vi "WS1050 36 DUT CP CV Sweep F12_B1 SubVI.vi"(0 "TMN DC\\CAP Data Log File Path":path=path "C:/WS1050 36 DUT Data", 1 "Test Program":string="WS1050 36 DUT CP CV Sweep SubVI", 3 "Lot#":string="WS1050", 4 "Wafer#":string="T7-EB", 5 "Board#":string="BRD5", 6 "Temp":string, 7 "error in (no error)":errorcluster, 8 "File Name":string="CYC_WS1050_T7_EB_65C_40V_25DC_EMPTY_BRD5_141017_1", 9 "Comment":string="CYC65C40V", 10 "Ke2400":refnum<visa-resource-name>="GPIB0::3::INSTR", 11 "PS1 Source":refnum<visa-resource-name>="GPIB0::5::INSTR", 12 "Serial Number":string[][](table)=[["DUT", "SN"], ["DUT1", "1"], ["DUT2", "2"], ["DUT3", "3"], ["DUT4", "4"], ["DUT5", "5"], ["DUT6", "6"], ["DUT7", "7"], ["DUT8", "8"], ["DUT9", "9"], ["DUT10", "10"], ["DUT11", "11"], ["DUT12", "12"], ["DUT13", "13"], ["DUT14", "14"], ["DUT15", "15"], ["DUT16", "16"], ["DUT17", "17"], ["DUT18", "18"], ["DUT19", "19"], ["DUT20", "20"], ["DUT21", "21"], ["DUT22", "22"], ["DUT23", "23"], ["DUT24", "24"], ["DUT25", "25"], ["DUT26", "26"], ["DUT27", "27"], ["DUT28", "28"], ["DUT29", "29"], ["DUT30", "30"], ["DUT31", "31"], ["DUT32", "32"], ["DUT33", "33"], ["DUT34", "34"], ["DUT35", "35"], ["DUT36", "36"]], 14 "CP Set to Run":dbl[][](array[numeric]), 16 "HD/Cycles Completed":string="Test Data", 18 "Ke2000":refnum<visa-resource-name>="GPIB0::9::INSTR") -> (13 "40V_1":string[][](table), 15 "40V_2":string[][](table), 17 "40V_3":string[][](table), 20 "Plot_1":dbl[][](graph) caption="(Y) Multi Plot 2", 21 "Plot_2":dbl[][](graph) caption="(Y) Multi Plot 2", 22 "Ke2400 Out":refnum<visa-resource-name>="GPIB0::3::INSTR", 23 "Plot_3":dbl[][](graph) caption="(Y) Multi Plot 2", 24 "CP Voltage":string, 25 "PS1 Out":refnum<visa-resource-name>, 26 "Ke2000 Out":refnum<visa-resource-name>="GPIB0::9::INSTR", 27 "error out":errorcluster)   [LabVIEW 2012]
uses:
  WS_VCAP Driver 029/Source/WSVCAP Shell/Type Defs/WSVCAP SHL I2C DUT Mask Mode Enum.ctl
panel:
  in  "Reg1_Bit Cntrl":string[](array[string])=["01", "02", "04", "08", "10", "20", "40", "80", "03", "06", "0C", "D8", "33", "66", "CC", "07", "0E", "1C", "38", "70", "E0", "0F", "1E", "3C", "78", "F0", "1F", "3E", "7C", "F8", "3F", "7E", "FC", "7F", "FE", "FD", "FB", "F7", "EF", "DF", "BF", "7F", "FC", "F9", "F3", "E7", "CF", "9F", "3F", "F8", "F1", "E3", "C7", "8F", "1F", "F0", "E1", "C3", "87", "0F", "E0", "C1", "83", "07", "C0", "81", "03", "AA", "55", "00"]
  out "date string":string="5/19/2014"
  in  "VPI_Cmd":string[](array[string])=["00", "3B", "00"]
  in  "VPI Name":string[](array[string])=["All_Drivers OFF", "All Drivers ON", "All Drivers OFF2"]
  in  "Tab Control":T1(tab)
  in  "Set VDD":dbl=3.7 format="%.3g"
  in  "Clock Rate (Hz)":dbl=1000000.0 caption="Meas Speed" format="%.1p Hz"
  out "AR  Measurent(Hz)":dbl
  in  "RFFE Slave Address":u8=7 caption="Slave Address" format="0x%02x"
  in  "CP VPI":i32(ring) items=["CP HDC 35V", "CP HDC 40.25V", "CP HDC 27.5V", "CP HDC 30.5V", "CP HDC 44V"]
  in  "Control Panel":T2={"CP C-V \nSweep"=TRUE, "HD/CYC"=FALSE, "E-CAL"=FALSE, "DVA"=FALSE, "VPI"=FALSE, "VSA"=FALSE, "HS"=FALSE}
  out "CP C-V Sweep":bool
  out "HD/CYC":bool
  out "E-CAL":bool
  out "DVA":bool
  out "VPI":bool
  out "VSA":bool
  out "HS":bool
  in  "Freq(Hz)":string="12K"
  in  "Test Sequences":i32(ring) items=["C1_C2_C3", "C2_C1_C3", "C3_C2_C1"]
  in  "WS1050/51":bool=TRUE
  in  "CP with DVA ON":i32(ring) items=["CP HDC 35V", "CP HDC 40.25V", "CP HDC 27.5V", "CP HDC 30.5V", "CP HDC 44V"]
  in  "% Duty Cycle":string="NA"
  in  "Cmin/Act":bool=TRUE
  in  "Current Input":string="71.772763E+0"
  out "NOM IDD OFF(uA)":string
  out "No of HD/Cycle\nCompleted":i32
  out "Loop \ncompleted":i32=1
  out "Previous Time":string="12:20:26 PM"
  out "STATUS":string="Idle...."
  out "Total Delta C2(pF)":string[](array[string])
  out "Total Delta C1(pF)":string[](array[string])
  out "Total Delta C3(pF)":string[](array[string])
  out "RB Reg for HD/Cycle":string[](array[string])
  out "VPI C2":string[][](table)
  out "VPI C3":string[][](table)
  out "NOM IDD ON (uA)":string
  out "IDD_HD/CYC (uA)":string="164.601255E+0"
  out "IDD Stdby(uA)":string="2.606990E+0"
  out "VPI C1":string[][](table)
  out "Loops Run":i64
  out "VSA_V1":string[][](table)
  out "VSA_V2":string[][](table)
  out "VSA_V3":string[][](table)
  in  "VSA Voltage(V)":dbl[](array[numeric])=[-10.0, 0.0, 10.0]
  in  "X Repeat":i32=100
  out "% Delta C_T0":string[][](array[string])
  out "% Delta C":string[][](array[string])
  out "EFuse RB T0":string[](array[string])
  out "Current EFuse Read back":string[](array[string])
  out "EFuse Readback Status":bool[](array[boolean])
  in  "DeltaC Target Setting(pF)":dbl=7.375
  in  "Debug":bool
  in  "No of Rows\nFrom Spread Sheet":i32
  in  "Plot Delta Cmin":bool=TRUE
  in  "Plot":T3(ring)
  in  "Bank1":i32(ring)=6 items=["C1", "C2", "C3", "D_C1", "D_C2", "D_C3", "D_B1_C1", "D_B1_C2", "D_B1_C3"]
  in  "Bank2":i32(ring)=7 items=["C1", "C2", "C3", "D_C1", "D_C2", "D_C3", "D_B1_C1", "D_B1_C2", "D_B1_C3"]
  in  "Bank3":i32(ring)=8 items=["C1", "C2", "C3", "D_C1", "D_C2", "D_C3", "D_B1_C1", "D_B1_C2", "D_B1_C3"]
  # "Company:  WiSpry Inc\n20 Fairbanks Ste 198 Irvine CA 92618\n\nAuthor:  Andy V Tran\nCreated:  08/21/2015\nLabVIEW 2012 Pro\nTest Program:  WS1050 36 DUT CP CV Sweep SubVI\nFPGA: WS_VCAP Driver 029"
  # "Note for HD Duty Cycle:\n1.  Set time to start HD_DC (Min), default is 259200 (6 months) \n2.  Set Time for Duty Cycle ON/OFF, default setting is 2 minutes\n3.  No of Loops to RP = 3600s/(Time ALL ON(s) + Time ALL + OFF(s))\n4.  Set X Repeat = no of runs, default is 100 runs\n5.  Set TTF Completed to stop the test.\n\nVer 1.1 updated based on Ver1.0:\n1.  Updated the control panel ( CP C-V Sweep was set \"Yes\" by default)\n2.  CP Voltage sweep should be set up from look up table."
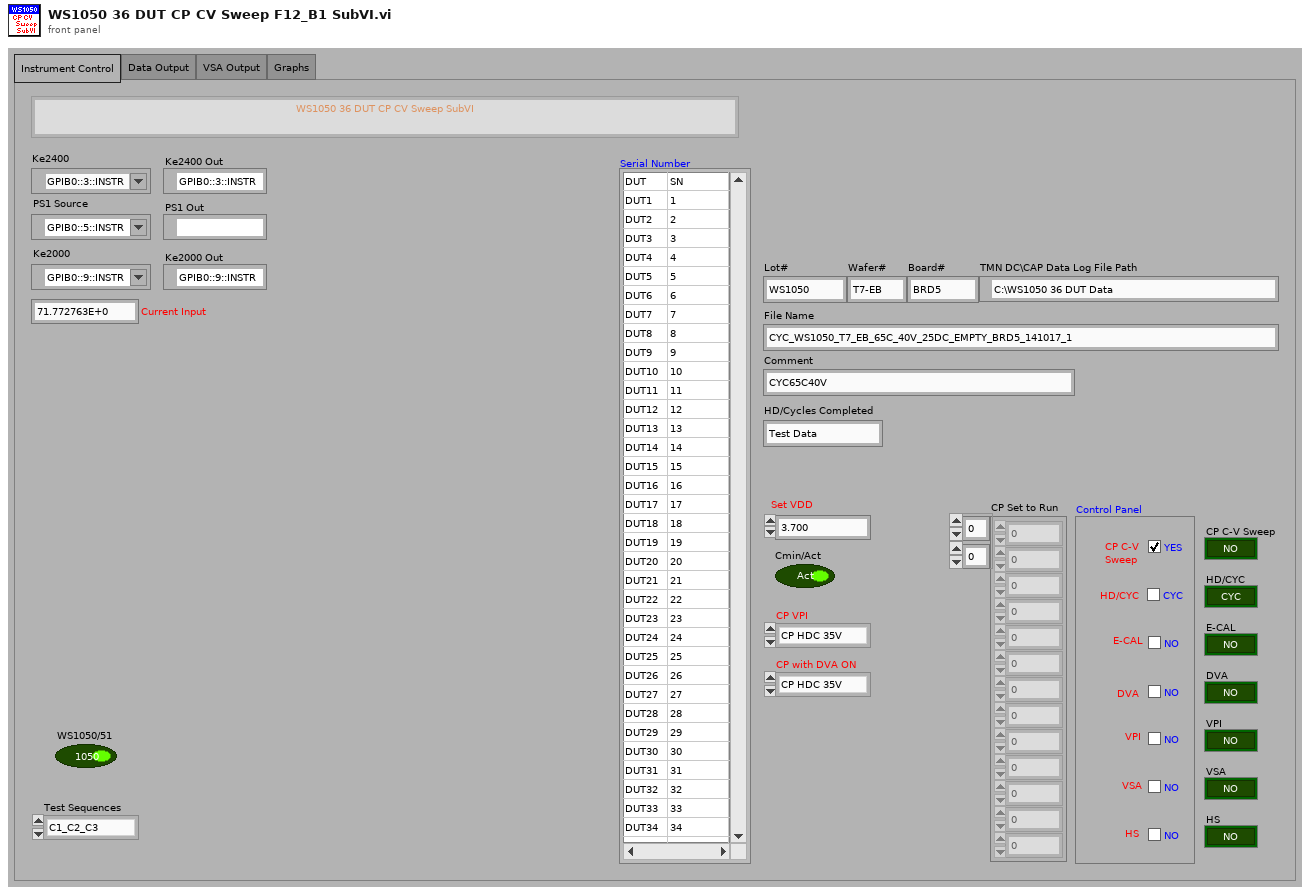
[diagram p1: front panel]
types:
  T1 = enum32{"Instrument Control", "Data Output", "VSA Output", "Graphs"}
  T2 = cluster{"CP C-V \nSweep":bool, "HD/CYC":bool, "E-CAL":bool, "DVA":bool, "VPI":bool, "VSA":bool, "HS":bool}
  T3 = enum16{"ALL DUTs", "DUT 01", "DUT 02", "DUT 03", "DUT 04", "DUT 05", "DUT 06", "DUT 07", "DUT 08", "DUT 09", "DUT 10", "DUT 11", "DUT 12", "DUT 13", "DUT 14", "DUT 15", "DUT 16", "DUT 17", "DUT 18", "DUT 19", "DUT 20", "DUT 21", "DUT 22", "DUT 23", "DUT 24", "DUT 25", "DUT 26", "DUT 27", "DUT 28", "DUT 29", "DUT 30", "DUT 31", "DUT 32", "DUT 33", "DUT 34", "DUT 35", "DUT 36"}
  T4 = typedef "WSVCAP SHL I2C DUT Mask Mode Enum.ctl" = enum16{"Custom", "C1", "C2", "C3", "All"}
  T5 = cluster{"Test Program ":string, "Comment":string, "Data Out":string, "Data Out":string, "CP Voltage":string, string, "% Duty Cycle":string, "CP Voltage":string, "string":string, "Freq(Hz)":string, "Board#":string}
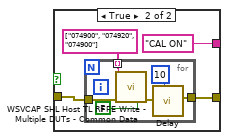
[diagram p3: hidden frame]
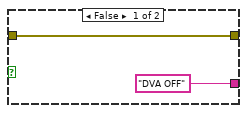
[diagram p4: hidden frame]
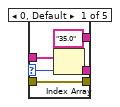
[diagram p5: hidden frame]
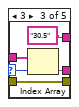
[diagram p6: hidden frame]
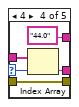
[diagram p7: hidden frame]
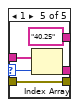
[diagram p8: hidden frame]
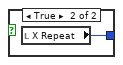
[diagram p9: hidden frame]
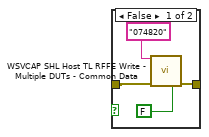
[diagram p10: hidden frame]
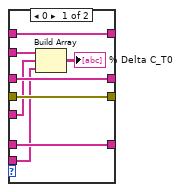
[diagram p11: hidden frame]
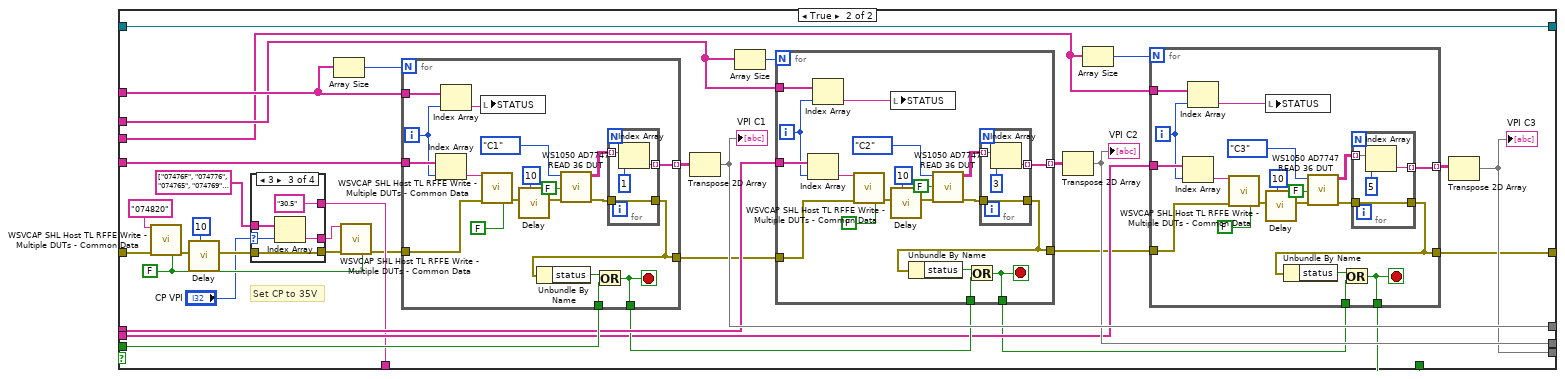
[diagram p12: hidden frame]
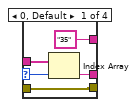
[diagram p13: hidden frame]
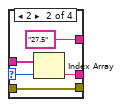
[diagram p14: hidden frame]
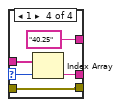
[diagram p15: hidden frame]
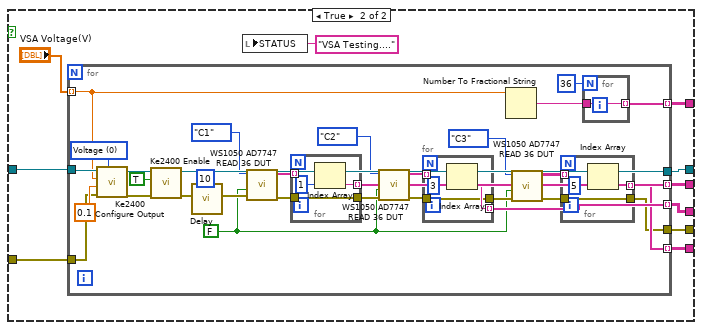
[diagram p17: hidden frame]
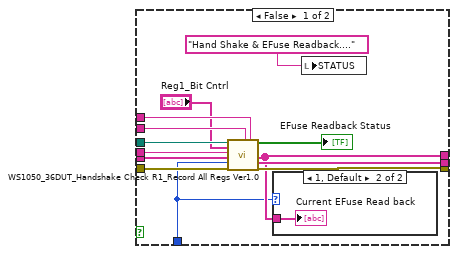
[diagram p18: hidden frame]
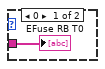
[diagram p19: hidden frame]
diagram:
  n1 = call "WSVCAP SHL Host TL RFFE Configure.vi"("RFFE Slave Address"="RFFE Slave Address", "Clock Rate (Hz)"="Clock Rate (Hz)", "error in"="error in (no error)") -> ("error out"=w4:errorcluster)  [unwired: 11 in, 1 out]
  n2 = call "Control Panel.vi"("error in (no error)"=w4, "Control Panel"="Control Panel") -> ("error out"=w12:errorcluster, "VPI"=w8:bool, "DVA"=w9:bool, "E-CAL"=w10:bool, "VSA"=w7:bool, "HD/CYC"=w11:bool, "HS"=w6:bool, "Verify Socket"=w1:bool)  [unwired: 2 in]
  "CP C-V Sweep" <- w1
  "E-CAL" <- w10
  "VPI" <- w8
  "VSA" <- w7
  "HS" <- w6
  "HD/CYC" <- w11
  "DVA" <- w9
  n3 = case shown="True" w1 {
    tunnel: w12 -> [w26 w28]
    tunnel: [w26 w32] -> w15
    tunnel: "CP Set to Run" -> [_ w76]
    tunnel: "PS1 Source" -> [w24 w29]
    tunnel: "Ke2000" -> [w25 w72]
    tunnel: [w25 w75] -> w22
    tunnel: [w24 w33] -> w21
    tunnel: "Ke2400" -> [w23 w69]
    tunnel: [w23 w66] -> w16
    tunnel: "RFFE Slave Address" -> [_ w64]
    tunnel: w11 -> [_ w43]
    tunnel: w10 -> [_ w42]
    tunnel: w9 -> [_ w27]
    tunnel: w8 -> [_ w41]
    tunnel: w7 -> [_ w40]
    tunnel: w6 -> [_ w39]
    tunnel: "Clock Rate (Hz)" -> [_ w31]
    frame False {
    }
    frame True {
      w30 = u32 1 ("milliseconds to wait")
      # "VSA"
      # "HS"
      # "HD/CYC"
      # "DVA"
      # "E-CAL"
      # "VPI"
      n4 = call "WSVCAP SHL Host TL RFFE Write - Multiple DUTs - Common Data.vi"("Data Out"="074000", "error in"=w28, "Log (T)"=FALSE) -> ("error out"=w74:errorcluster)  [unwired: 12 in]
      n5 = call "Delay.vi"("milliseconds to wait"=u32 100, "error in (no error)"=w74) -> ("error out"=w73:errorcluster)  [unwired: 9 in]
      n6 = call "Ke2000 Single Reading.vi"("error in (no error)"=w73, "VISA resource name"=w72) -> ("error out"=w54:errorcluster, "VISA resource name out"=w71:refnum<visa-resource-name>, "uA"=w56:string)  [unwired: 5 in, 2 out]
      n7 = call "Substration.vi"("error in (no error)"=w54, "Input2"="Current Input", "Input1"=w56) -> ("error out"=w36:errorcluster, "In1 - In2"=w55:string)  [unwired: 7 in]
      "IDD Stdby(uA)" <- w55
      n8 = case shown="False" w43 {
        tunnel: [1 ("X Repeat") w133] -> w65
        frame False {
        }
        frame True {
          n9 = local read "X Repeat"() -> (w133:i32)
        }
      }
      n10 = call "WSVCAP SHL Host TL RFFE Write - Multiple DUTs - Common Data.vi"("Data Out"="074040", "error in"=w36, "Log (T)"=FALSE) -> ("error out"=w35:errorcluster)  [unwired: 12 in]
      n11 = call "Delay.vi"("milliseconds to wait"=w30, "error in (no error)"=w35) -> ("error out"=w62:errorcluster)  [unwired: 9 in]
      n12 = case shown="True" w27 {
        tunnel: w62 -> [w94 w104]
        tunnel: [w94 w102] -> w60
        tunnel: ["DVA OFF" ("Data Out") "DVA ON" ("Data Out")] -> w61
        frame False {
        }
        frame True {
          n13 = call "WSVCAP SHL Host TL RFFE Write - Multiple DUTs - Common Data.vi"("Data Out"="074800", "error in"=w104, "Log (T)"=FALSE) -> ("error out"=w100:errorcluster)  [unwired: 12 in]
          n14 = case shown="2" "CP with DVA ON" {
            selector: "CP with DVA ON" -> [w110 w115 w120 w125 w129]
            tunnel: string[] ["07442F", "074436", "074428", "074429", "07443B"] -> [w111 w116 w121 w126 w131]
            tunnel: [w109 w114 w119 w124 w130] -> w96
            tunnel: ["35.0" ("Data Out") "29.75" ("Data Out") "30.5" ("Data Out") "44.0" ("Data Out") "40.25" ("Data Out")] -> _
            tunnel: w100 -> [w107 w112 w117 w122 w127]
            tunnel: [w107 w112 w117 w122 w127] -> w99
            frame 0, Default {
              n15 = Index Array(array=w111, index=w110) -> (element=w109:string)
            }
            frame 2 {
              n16 = Index Array(array=w116, index=w115) -> (element=w114:string)
            }
            frame 3 {
              n17 = Index Array(array=w121, index=w120) -> (element=w119:string)
            }
            frame 4 {
              n18 = Index Array(array=w126, index=w125) -> (element=w124:string)
            }
            frame 1 {
              n19 = Index Array(array=w131, index=w129) -> (element=w130:string)
            }
          }
          n20 = call "WSVCAP SHL Host TL RFFE Write - Multiple DUTs - Common Data.vi"("Data Out"=w96, "error in"=w99, "Log (T)"=FALSE) -> ("error out"=w102:errorcluster)  [unwired: 12 in]
        }
      }
      n21 = for {
        N: 36 -> [_]
        tunnel: "Serial Number" -> [w81]
        tunnel: [w79] -> w45 mode=indexing
        i -> [w78]
        n22 = Increment(x=w78) -> (x+1=w77:i32)
        n23 = Index Array(array=w81, index (row)=w77, index (col)=1 ("disabled index (col)")) -> (element=w79:string)
      }
      n24 = Not(x=w39) -> (.not. x?=w44:bool)
      n25 = Number To Fractional String(number="Set VDD", precision (6)=i16 2) -> (F-format string=w58:string)  [unwired: 2 in]
      n26 = call "Delay.vi"("milliseconds to wait"=w30, "error in (no error)"=w60) -> ("error out"=w51:errorcluster)  [unwired: 9 in]
      n27 = case shown="False" w42 {
        tunnel: w51 -> [w82 w85]
        tunnel: [w82 w84] -> w50
        tunnel: ["CAL OFF" ("Data Out") "CAL ON" ("Data Out")] -> w52
        frame False {
        }
        frame True {
          n28 = for {
            tunnel: string[] ["074900", "074920", "074900"] -> [w93] mode=indexing
            tunnel: w85 -> [w90]
            tunnel: [w89] -> w84
            n29 = call "WSVCAP SHL Host TL RFFE Write - Multiple DUTs - Common Data.vi"("Data Out"=w93, "error in"=w90, "Log (T)"=FALSE) -> ("error out"=w92:errorcluster)  [unwired: 12 in]
            n30 = call "Delay.vi"("milliseconds to wait"=u32 10, "error in (no error)"=w92) -> ("error out"=w89:errorcluster)  [unwired: 9 in]
          }
        }
      }
      n31 = for {
        N: w65 -> [_]
        tunnel: w76 -> [w162]
        tunnel: [w158] -> w75
        tunnel: w55 -> [w157]
        tunnel: w71 -> [w156]
        tunnel: "TMN DC\\CAP Data Log File Path" -> [w155]
        tunnel: w69 -> [w153]
        tunnel: [w152] -> w67
        tunnel: w29 -> [w137]
        tunnel: w64 -> [w148]
        tunnel: w61 -> [w147]
        tunnel: w58 -> [w146]
        tunnel: [w145] -> w53
        tunnel: w52 -> [w144]
        tunnel: w50 -> [w143]
        tunnel: w27 -> [w142]
        tunnel: w41 -> [w141]
        tunnel: w44 -> [w140]
        tunnel: w40 -> [w139]
        tunnel: w45 -> [w138]
        tunnel: [w137] -> w33
        tunnel: "Current Input" -> [w136]
        tunnel: w31 -> [w134]
        stop <- w135 stop-if-true
        (unwired) u64 0
        n32 = while {
          tunnel: w162 -> [w180]
          tunnel: w155 -> [w381]
          tunnel: "Lot#" -> [w380]
          tunnel: "Wafer#" -> [w379]
          tunnel: w138 -> [w378]
          tunnel: "Test Program" -> [w377]
          tunnel: w138 -> [w376]
          tunnel: "Comment" -> [w375]
          tunnel: "Lot#" -> [w374]
          tunnel: "Wafer#" -> [w373]
          tunnel: w156 -> [w370]
          tunnel: [w372] -> w158
          tunnel: w157 -> [w369]
          tunnel: w153 -> [w367]
          tunnel: [w366] -> w152
          tunnel: [w291] -> w149
          tunnel: w148 -> [w290]
          tunnel: w147 -> [w240]
          tunnel: w146 -> [w238]
          tunnel: [w220] -> w145
          tunnel: w144 -> [w225]
          tunnel: w143 -> [w181]
          tunnel: w142 -> [w224]
          tunnel: w141 -> [w217]
          tunnel: w140 -> [w212]
          tunnel: w139 -> [w206]
          tunnel: w136 -> [w166]
          tunnel: w134 -> [w165]
          i -> [w185]
          stop <- w320 stop-if-true
          n33 = Array Size(array=w180) -> (size(s)=w179:i32[])
          n34 = Index Array(array=w180, index (row)=w185, index (col)=0 ("disabled index (col)")) -> (element=w177:dbl)
          n35 = Index Array(array=w179, index=0) -> (element=w168:i32)
          n36 = call "CP_Cmd_Setting.vi"("error in (no error)"=w181, "Input"=w177) -> ("error out"=w184:errorcluster, "CP Voltage"=w182:string, "Send Cmd"=w183:string)  [unwired: 6 in, 1 out]
          "CP Voltage" <- w182
          n37 = To Quad Integer(1:w168) -> (0:w167:i64)
          n38 = flat-sequence {
            tunnel: [w434] -> w365
            tunnel: w370 -> [w423]
            tunnel: w369 -> [w435]
            tunnel: [w435] -> w364
            tunnel: [w400] -> w363
            tunnel: [w397] -> w362
            tunnel: w184 -> [w432]
            tunnel: w185 -> [w382]
            tunnel: [w382] -> w319
            tunnel: ["Temp"] -> w314
            tunnel: [w405] -> w309
            tunnel: [w404] -> w308
            tunnel: [w403] -> w307
            tunnel: [w409] -> w297
            tunnel: [w406] -> w296
            tunnel: w290 -> [w431]
            tunnel: [w431] -> w289
            tunnel: [w408] -> w277
            tunnel: [w407] -> w253
            tunnel: [w383] -> w241
            tunnel: w183 -> [w429]
            tunnel: ["% Duty Cycle"] -> w237
            tunnel: [w390] -> w229
            tunnel: w217 -> [w418]
            tunnel: [w418] -> w216
            tunnel: w212 -> [w417]
            tunnel: [w417] -> w211
            tunnel: w206 -> [w416]
            tunnel: [w416] -> w205
            tunnel: [w412] -> w200
            tunnel: ["WS1050/51"] -> w194
            tunnel: ["Cmin/Act"] -> w190
            tunnel: w167 -> [w388]
            tunnel: w177 -> [w389]
            tunnel: [w388] -> w176
            tunnel: w166 -> [w387]
            tunnel: w165 -> [w383]
            tunnel: [w487] -> w288
            tunnel: w365 -> [w490]
            tunnel: w364 -> [w493]
            tunnel: w363 -> [w489]
            tunnel: w362 -> [w488]
            tunnel: [w478] -> w287
            tunnel: [w493] -> w286
            tunnel: [w489] -> w285
            tunnel: [w488] -> w284
            tunnel: w319 -> [w492]
            tunnel: [w492] -> w283
            tunnel: w314 -> [w491]
            tunnel: [w491] -> w282
            tunnel: [w490] -> w281
            tunnel: w309 -> [w486]
            tunnel: w308 -> [w471]
            tunnel: w307 -> [w472]
            tunnel: [w483] -> w280
            tunnel: w297 -> [w485]
            tunnel: w296 -> [w483]
            tunnel: [w479] -> w279
            tunnel: w289 -> [w484]
            tunnel: [w469] -> w278
            tunnel: w277 -> [w469]
            tunnel: [w471] -> w276
            tunnel: w253 -> [w470]
            tunnel: [w470] -> w252
            tunnel: [w472] -> w250
            tunnel: w241 -> [w482]
            tunnel: [w481] -> w230
            tunnel: w229 -> [w481]
            tunnel: w216 -> [w477]
            tunnel: [w477] -> w215
            tunnel: w211 -> [w476]
            tunnel: [w476] -> w210
            tunnel: w205 -> [w475]
            tunnel: [w475] -> w204
            tunnel: w200 -> [w474]
            tunnel: [w473] -> w199
            tunnel: w194 -> [w467]
            tunnel: [w467] -> w193
            tunnel: w190 -> [w466]
            tunnel: [w466] -> w189
            tunnel: w176 -> [w465]
            tunnel: [w465] -> w175
            tunnel: w288 -> [w532]
            tunnel: [w531] -> w275
            tunnel: w287 -> [w523]
            tunnel: [w523] -> w272
            tunnel: w286 -> [w542]
            tunnel: [w542] -> w270
            tunnel: w285 -> [w541]
            tunnel: [w541] -> w268
            tunnel: w284 -> [w540]
            tunnel: [w540] -> w266
            tunnel: w283 -> [w539]
            tunnel: [w539] -> w264
            tunnel: w282 -> [w538]
            tunnel: [w538] -> w262
            tunnel: w281 -> [w537]
            tunnel: [w537] -> w260
            tunnel: w280 -> [w536]
            tunnel: [w536] -> w258
            tunnel: [w528] -> w256
            tunnel: w279 -> [w527]
            tunnel: w278 -> [w534]
            tunnel: w276 -> [w533]
            tunnel: w252 -> [w520]
            tunnel: [w520] -> w251
            tunnel: w250 -> [w522]
            tunnel: [w522] -> w249
            tunnel: [w529] -> w248
            tunnel: [w530] -> w231
            tunnel: w230 -> [w530]
            tunnel: w215 -> [w526]
            tunnel: [w526] -> w214
            tunnel: w210 -> [w525]
            tunnel: [w525] -> w209
            tunnel: w204 -> [w524]
            tunnel: [w524] -> w203
            tunnel: w199 -> [w521]
            tunnel: [w521] -> w196
            tunnel: w193 -> [w518]
            tunnel: [w518] -> w192
            tunnel: w189 -> [w517]
            tunnel: [w517] -> w188
            tunnel: w175 -> [w516]
            tunnel: [w516] -> w174
            tunnel: w275 -> [w582]
            tunnel: [w581] -> w274
            tunnel: [w577] -> w273
            tunnel: w272 -> [w571]
            tunnel: [w571] -> w271
            tunnel: w270 -> [w593]
            tunnel: [w593] -> w269
            tunnel: w268 -> [w592]
            tunnel: [w592] -> w267
            tunnel: w266 -> [w591]
            tunnel: [w591] -> w265
            tunnel: w264 -> [w590]
            tunnel: [w590] -> w263
            tunnel: w262 -> [w589]
            tunnel: [w589] -> w261
            tunnel: w260 -> [w588]
            tunnel: [w588] -> w259
            tunnel: w258 -> [w587]
            tunnel: [w587] -> w257
            tunnel: w256 -> [w586]
            tunnel: [w586] -> w255
            tunnel: [w569] -> w254
            tunnel: w251 -> [w584]
            tunnel: w249 -> [w583]
            tunnel: w248 -> [w576]
            tunnel: ["DeltaC Target Setting(pF)"] -> w239
            tunnel: [w579] -> w232
            tunnel: w231 -> [w579]
            tunnel: w224 -> [w578]
            tunnel: [w578] -> w223
            tunnel: w214 -> [w575]
            tunnel: [w575] -> w213
            tunnel: w209 -> [w574]
            tunnel: [w574] -> w208
            tunnel: w203 -> [w573]
            tunnel: [w573] -> w202
            tunnel: w196 -> [w572]
            tunnel: [w569] -> w195
            tunnel: w192 -> [w568]
            tunnel: [w568] -> w191
            tunnel: w188 -> [w567]
            tunnel: [w567] -> w187
            tunnel: w174 -> [w566]
            tunnel: [w566] -> w173
            tunnel: [w671] -> w361
            tunnel: [w640] -> w360
            tunnel: w274 -> [w674]
            tunnel: w273 -> [w651]
            tunnel: [w660] -> w359
            tunnel: [w651] -> w358
            tunnel: [w673] -> w357
            tunnel: [w672] -> w356
            tunnel: w271 -> [w660]
            tunnel: w269 -> [w670]
            tunnel: [w670] -> w355
            tunnel: w267 -> [w666]
            tunnel: [w666] -> w354
            tunnel: w265 -> [w665]
            tunnel: [w665] -> w353
            tunnel: w263 -> [w661]
            tunnel: [w661] -> w318
            tunnel: w261 -> [w669]
            tunnel: [w669] -> w313
            tunnel: w259 -> [w668]
            tunnel: [w667] -> w310
            tunnel: w257 -> [w663]
            tunnel: w255 -> [w659]
            tunnel: [w664] -> w306
            tunnel: [w662] -> w305
            tunnel: [w659] -> w300
            tunnel: w254 -> [w658]
            tunnel: [w648] -> w295
            tunnel: [w647] -> w294
            tunnel: [w646] -> w293
            tunnel: w239 -> [w657]
            tunnel: [w645] -> w233
            tunnel: w232 -> [w645]
            tunnel: [w644] -> w228
            tunnel: w223 -> [w643]
            tunnel: w213 -> [w638]
            tunnel: w208 -> [w637]
            tunnel: [w637] -> w207
            tunnel: w202 -> [w636]
            tunnel: [w636] -> w201
            tunnel: w195 -> [w633]
            tunnel: w191 -> [w632]
            tunnel: w187 -> [w621]
            tunnel: w173 -> [w620]
            tunnel: [w620] -> w172
            tunnel: w361 -> [w877]
            tunnel: [w877] -> w352
            tunnel: [w863] -> w351
            tunnel: [w876] -> w350
            tunnel: w360 -> [w875]
            tunnel: w359 -> [w874]
            tunnel: w358 -> [w873]
            tunnel: [w874] -> w349
            tunnel: [w873] -> w348
            tunnel: w357 -> [w872]
            tunnel: [w872] -> w347
            tunnel: w356 -> [w871]
            tunnel: [w871] -> w346
            tunnel: w355 -> [w870]
            tunnel: [w870] -> w345
            tunnel: w354 -> [w869]
            tunnel: [w869] -> w344
            tunnel: w353 -> [w868]
            tunnel: [w868] -> w343
            tunnel: w367 -> [w867]
            tunnel: [w865] -> w342
            tunnel: [w845] -> w341
            tunnel: [w846] -> w340
            tunnel: [w844] -> w339
            tunnel: w318 -> [w861]
            tunnel: [w861] -> w317
            tunnel: w313 -> [w860]
            tunnel: [w860] -> w312
            tunnel: w310 -> [w876]
            tunnel: w306 -> [w858]
            tunnel: w305 -> [w859]
            tunnel: [w859] -> w304
            tunnel: [w858] -> w302
            tunnel: w300 -> [w857]
            tunnel: [w857] -> w299
            tunnel: w295 -> [w843]
            tunnel: w294 -> [w842]
            tunnel: w293 -> [w841]
            tunnel: [w838] -> w292
            tunnel: [w843] -> w247
            tunnel: [w842] -> w245
            tunnel: [w841] -> w243
            tunnel: [w840] -> w234
            tunnel: w233 -> [w840]
            tunnel: w228 -> [w839]
            tunnel: [w839] -> w227
            tunnel: w207 -> [w838]
            tunnel: w201 -> [w837]
            tunnel: w172 -> [w836]
            tunnel: [w836] -> w171
            tunnel: w352 -> [w971]
            tunnel: [w971] -> w338
            tunnel: w351 -> [w992]
            tunnel: [w991] -> w337
            tunnel: w381 -> [w993]
            tunnel: w380 -> [w990]
            tunnel: w379 -> [w989]
            tunnel: w378 -> [w988]
            tunnel: [w987] -> w336
            tunnel: w350 -> [w981]
            tunnel: [w981] -> w335
            tunnel: w349 -> [w986]
            tunnel: w348 -> [w985]
            tunnel: [w986] -> w334
            tunnel: [w985] -> w333
            tunnel: [w979] -> w332
            tunnel: w347 -> [w984]
            tunnel: [w984] -> w331
            tunnel: w346 -> [w983]
            tunnel: [w983] -> w330
            tunnel: [w982] -> w329
            tunnel: w345 -> [w980]
            tunnel: w344 -> [w978]
            tunnel: w343 -> [w977]
            tunnel: "File Name" -> [w976]
            tunnel: w342 -> [w975]
            tunnel: [w975] -> w328
            tunnel: w341 -> [w974]
            tunnel: [w974] -> w327
            tunnel: [w973] -> w326
            tunnel: w340 -> [w973]
            tunnel: w339 -> [w972]
            tunnel: [w972] -> w325
            tunnel: w317 -> [w955]
            tunnel: [w955] -> w315
            tunnel: w312 -> [w969]
            tunnel: [w969] -> w311
            tunnel: w304 -> [w968]
            tunnel: [w968] -> w303
            tunnel: w302 -> [w967]
            tunnel: [w967] -> w301
            tunnel: w299 -> [w966]
            tunnel: [w966] -> w298
            tunnel: w292 -> [w965]
            tunnel: w247 -> [w964]
            tunnel: [w964] -> w246
            tunnel: w245 -> [w963]
            tunnel: [w963] -> w244
            tunnel: w243 -> [w962]
            tunnel: [w962] -> w242
            tunnel: w237 -> [w961]
            tunnel: [w961] -> w236
            tunnel: [w960] -> w235
            tunnel: w234 -> [w960]
            tunnel: w227 -> [w959]
            tunnel: [w959] -> w226
            tunnel: ["Freq(Hz)"] -> w198
            tunnel: ["Board#"] -> w197
            tunnel: w171 -> [w956]
            tunnel: [w956] -> w170
            tunnel: ["Debug"] -> w164
            tunnel: w338 -> [w1066]
            tunnel: w337 -> [w1065]
            tunnel: w381 -> [w1032]
            tunnel: w377 -> [w1060]
            tunnel: w376 -> [w1063]
            tunnel: w375 -> [w1059]
            tunnel: w374 -> [w1062]
            tunnel: w373 -> [w1058]
            tunnel: w336 -> [w1061]
            tunnel: [w1066] -> w322
            tunnel: [w1064] -> w323
            tunnel: w335 -> [w1056]
            tunnel: [w1056] -> w324
            tunnel: w334 -> [w1055]
            tunnel: w333 -> [w1043]
            tunnel: w332 -> [w1054]
            tunnel: w331 -> [w1053]
            tunnel: w330 -> [w1045]
            tunnel: w329 -> [w1052]
            tunnel: "File Name" -> [w1026]
            tunnel: w328 -> [w1051]
            tunnel: [w1051] -> w321
            tunnel: w327 -> [w1050]
            tunnel: w326 -> [w1049]
            tunnel: w325 -> [w1048]
            tunnel: [w1028] -> w316
            tunnel: w315 -> [w1028]
            tunnel: w311 -> [w1047]
            tunnel: w303 -> [w1046]
            tunnel: w301 -> [w1044]
            tunnel: w298 -> [w1015]
            tunnel: w246 -> [w1042]
            tunnel: w244 -> [w1041]
            tunnel: w242 -> [w1040]
            tunnel: w240 -> [w1039]
            tunnel: w225 -> [w1038]
            tunnel: w182 -> [w1037]
            tunnel: w238 -> [w1036]
            tunnel: w236 -> [w1035]
            tunnel: w235 -> [w1034]
            tunnel: w226 -> [w1033]
            tunnel: [w1030] -> w222
            tunnel: [w1023] -> w218
            tunnel: w198 -> [w1022]
            tunnel: w197 -> [w1020]
            tunnel: w170 -> [w1019]
            tunnel: [w1019] -> w169
            tunnel: w164 -> [w1017]
            tunnel: [w1085] -> w371
            tunnel: [w1086] -> w372
            tunnel: [w1087] -> w291
            tunnel: w324 -> [w1086]
            tunnel: w323 -> [w1079]
            tunnel: w322 -> [w1087]
            tunnel: w321 -> [w1080]
            tunnel: [w1080] -> w366
            tunnel: w316 -> [w1072]
            tunnel: [w1078] -> w219
            tunnel: w222 -> [w1077]
            tunnel: w218 -> [w1075]
            tunnel: w169 -> [w1074]
            tunnel: [w1071] -> w163
            frame #0 {
              w413 = FALSE ("Log (T)")
              n39 = call "WSVCAP SHL Host TL RFFE Write - Multiple DUTs - Common Data.vi"("Data Out"=w429, "error in"=w432, "Log (T)"=FALSE) -> ("error out"=w419:errorcluster)  [unwired: 12 in]
              n40 = for {
                tunnel: string[] ["0760", "0767", "0768"] -> [w457] mode=indexing
                tunnel: [w453] -> w421 mode=indexing
                tunnel: w419 -> [w451]
                tunnel: [w450] -> w420
                i -> [w456]
                n41 = call "Delay.vi"("milliseconds to wait"=u32 10, "error in (no error)"=w451) -> ("error out"=w458:errorcluster)  [unwired: 9 in]
                n42 = call "WSVCAP SHL Host TL RFFE Read - Multiple DUTs - Common Data.vi"("Data Out"=w457, "error in"=w458, "Log (T)"=FALSE) -> ("RFFE Data In"=w455:string[], "error out"=w450:errorcluster)  [unwired: 11 in]
                n43 = Index Array(array=w455, index=w456) -> (element=w452:string)
                n44 = String Subset(string=w452, offset (0)=0) -> (substring=w453:string)  [unwired: 1 in]
              }
              "RB Reg for HD/Cycle" <- w421
              n45 = call "Delay.vi"("milliseconds to wait"=u32 100, "error in (no error)"=w420) -> ("error out"=w425:errorcluster)  [unwired: 9 in]
              n46 = call "Ke2000 Single Reading.vi"("error in (no error)"=w425, "VISA resource name"=w423) -> ("error out"=w427:errorcluster, "VISA resource name out"=w402:refnum<visa-resource-name>, "uA"=w428:string)  [unwired: 5 in, 2 out]
              n47 = call "Substration.vi"("error in (no error)"=w427, "Input2"=w387, "Input1"=w428) -> ("error out"=w384:errorcluster, "In1 - In2"=→"IDD_HD/CYC (uA)":string)  [unwired: 7 in]
              n48 = call "CP_Cmd_Setting.vi"("error in (no error)"=w384, "Input"=w389) -> ("error out"=w392:errorcluster, "CP Voltage"=w390:string, "Send Cmd"=w391:string)  [unwired: 6 in, 1 out]
              n49 = call "WSVCAP SHL Host TL RFFE Write - Multiple DUTs - Common Data.vi"("Data Out"=w391, "error in"=w392, "Log (T)"=w413) -> ("error out"=w430:errorcluster)  [unwired: 12 in]
              n50 = flat-sequence {
                tunnel: w415 -> [w460]
                tunnel: [w460] -> w411
                frame #0 {
                  w461 = "0" ("NOM IDD OFF(uA)")
                  w462 = string[] []
                  w463 = string[][] []
                  n51 = local write "Total Delta C1(pF)"(w462) -> ()
                  n52 = local write "Total Delta C2(pF)"(w462) -> ()
                  n53 = local write "Total Delta C3(pF)"(w462) -> ()
                  n54 = local write "Current EFuse Read back"(w462) -> ()
                  n55 = local write "NOM IDD ON (uA)"(w461) -> ()
                  n56 = local write "NOM IDD OFF(uA)"(w461) -> ()
                  n57 = local write "VSA_V3"(w463) -> ()
                  n58 = local write "VSA_V1"(w463) -> ()
                  n59 = local write "VSA_V2"(w463) -> ()
                  n60 = local write "VPI C1"(w463) -> ()
                  n61 = local write "VPI C2"(w463) -> ()
                  n62 = local write "VPI C3"(w463) -> ()
                  n63 = local write "% Delta C"(w463) -> ()
                  n64 = local write "40V_3"(w463) -> ()
                  n65 = local write "40V_2"(w463) -> ()
                  n66 = local write "40V_1"(w463) -> ()
                }
              }
              n67 = call "Delay.vi"("milliseconds to wait"=u32 10, "error in (no error)"=w430) -> ("error out"=w395:errorcluster)  [unwired: 9 in]
              n68 = for {
                tunnel: [w448] -> w434
                tunnel: [w447] -> w415
                tunnel: w413 -> [w446]
                tunnel: w402 -> [w445]
                tunnel: w395 -> [w441]
                tunnel: string[] ["0702013B3B3B", "070201000000"] -> [w438] mode=indexing
                tunnel: [w437] -> w398 mode=indexing
                tunnel: w387 -> [w436]
                n69 = call "WSVCAP SHL Host TL RFFE Write - Multiple DUTs - Common Data.vi"("Data Out"=w438, "error in"=w441, "Log (T)"=w446) -> ("error out"=w442:errorcluster)  [unwired: 12 in]
                n70 = call "Delay.vi"("milliseconds to wait"=u32 100, "error in (no error)"=w442) -> ("error out"=w443:errorcluster)  [unwired: 9 in]
                n71 = call "Ke2000 Single Reading.vi"("error in (no error)"=w443, "VISA resource name"=w445) -> ("error out"=w440:errorcluster, "VISA resource name out"=w448:refnum<visa-resource-name>, "uA"=w439:string)  [unwired: 5 in, 2 out]
                n72 = call "Substration.vi"("error in (no error)"=w440, "Input2"=w436, "Input1"=w439) -> ("error out"=w447:errorcluster, "In1 - In2"=w437:string)  [unwired: 7 in]
              }
              n73 = Index Array(array=w398, index=0) -> (element=w400:string)
              n74 = Index Array(array=w398, index=1) -> (element=w397:string)
              n75 = call "Multi Dut Cmd_Header Setting F12_B1.vi"("WS1050/51"="WS1050/51", "Cmin/Act"="Cmin/Act", "Test Seq"="Test Sequences", "error in (no error)"=w411) -> ("Name 1"=w409:string[], "Name 2"=w408:string[], "Name Header"=w406:string[], "Name 3"=w407:string[], "Cmd 3"=w403:string[], "Cmd 1"=w405:string[], "Cmd 2"=w404:string[], "error out"=w412:errorcluster)  [unwired: 2 in, 2 out]
              "Loops Run" <- w388
            }
            frame #1 {
              w473 = FALSE ("Log (T)")
              n76 = call "WSVCAP SHL Host TL RFFE Configure.vi"("RFFE Slave Address"=w484, "Clock Rate (Hz)"=w482, "error in"=w474) -> ("Actual Rate (Hz)"=→"AR  Measurent(Hz)":dbl, "error out"=w480:errorcluster)  [unwired: 11 in]
              n77 = Array Size(array=w485) -> (size(s)=w494:i32)
              n78 = for {
                N: w494 -> [_]
                tunnel: w486 -> [w511]
                tunnel: [w495] -> w487
                tunnel: [w507] -> w468 mode=indexing
                tunnel: w485 -> [w509]
                tunnel: w480 -> [w497]
                tunnel: [w499] -> w479
                tunnel: w473 -> [w498]
                i -> [w506]
                stop <- w495 stop-if-true
                n79 = Index Array(array=w511, index=w506) -> (element=w510:string)
                n80 = Index Array(array=w509, index=w506) -> (element=w508:string)
                n81 = local write "STATUS"(w508) -> ()
                n82 = call "WSVCAP SHL Host TL RFFE Write - Multiple DUTs - Common Data.vi"("Data Out"=w510, "error in"=w497, "Log (T)"=FALSE) -> ("error out"=w501:errorcluster)  [unwired: 12 in]
                n83 = call "Delay.vi"("milliseconds to wait"=u32 10, "error in (no error)"=w501) -> ("error out"=w505:errorcluster)  [unwired: 9 in]
                n84 = call "WS1050 AD7747 READ 36 DUT.vi"("error in"=w505, "Log (T)"=w498, "DUT Mask Mode (All)"=WSVCAP_SHL_I2C_DUT_Mask_Mode_Enum."C1") -> ("error out"=w503:errorcluster, "AD7747 Values"=w504:string[][])  [unwired: 7 in]
                n85 = for {
                  tunnel: w504 -> [w514] mode=indexing
                  tunnel: w503 -> [w515]
                  tunnel: [w515] -> w499
                  tunnel: [w512] -> w507 mode=indexing
                  n86 = Index Array(array=w514, index=1) -> (element=w512:string)
                }
                n87 = Unbundle By Name(w499) -> ("status"=w495:bool)
              }
              n88 = Transpose 2D Array(2D array=w468) -> (transposed array=w478:string[][])
              "40V_1" <- w478
              "NOM IDD ON (uA)" <- w489
              "NOM IDD OFF(uA)" <- w488
            }
            frame #2 {
              n89 = Array Size(array=w534) -> (size(s)=w535:i32)
              n90 = for {
                N: w535 -> [_]
                tunnel: w533 -> [w561]
                tunnel: w532 -> [w559]
                tunnel: [w558] -> w531
                tunnel: [w554] -> w519 mode=indexing
                tunnel: w534 -> [w556]
                tunnel: w527 -> [w544]
                tunnel: [w546] -> w529
                tunnel: w521 -> [w545]
                i -> [w553]
                stop <- w558 stop-if-true
                n91 = Index Array(array=w561, index=w553) -> (element=w557:string)
                n92 = Index Array(array=w556, index=w553) -> (element=w555:string)
                n93 = call "WSVCAP SHL Host TL RFFE Write - Multiple DUTs - Common Data.vi"("Data Out"=w557, "error in"=w544, "Log (T)"=FALSE) -> ("error out"=w548:errorcluster)  [unwired: 12 in]
                n94 = local write "STATUS"(w555) -> ()
                n95 = call "Delay.vi"("milliseconds to wait"=u32 10, "error in (no error)"=w548) -> ("error out"=w552:errorcluster)  [unwired: 9 in]
                n96 = call "WS1050 AD7747 READ 36 DUT.vi"("error in"=w552, "Log (T)"=w545, "DUT Mask Mode (All)"=WSVCAP_SHL_I2C_DUT_Mask_Mode_Enum."C2") -> ("error out"=w550:errorcluster, "AD7747 Values"=w551:string[][])  [unwired: 7 in]
                n97 = for {
                  tunnel: w551 -> [w564] mode=indexing
                  tunnel: w550 -> [w565]
                  tunnel: [w565] -> w546
                  tunnel: [w562] -> w554 mode=indexing
                  n98 = Index Array(array=w564, index=3) -> (element=w562:string)
                }
                n99 = Unbundle By Name(w546) -> ("status"=w560:bool)
                n100 = Or(x=w560, y=w559) -> (x .or. y?=w558:bool)
              }
              n101 = Transpose 2D Array(2D array=w519) -> (transposed array=w528:string[][])
              "40V_2" <- w528
            }
            frame #3 {
              n102 = Array Size(array=w584) -> (size(s)=w585:i32)
              n103 = for {
                N: w585 -> [_]
                tunnel: w583 -> [w612]
                tunnel: w582 -> [w610]
                tunnel: [w609] -> w581
                tunnel: [w605] -> w570 mode=indexing
                tunnel: w584 -> [w607]
                tunnel: w576 -> [w595]
                tunnel: [w597] -> w569
                tunnel: w572 -> [w596]
                i -> [w604]
                stop <- w609 stop-if-true
                n104 = Index Array(array=w612, index=w604) -> (element=w608:string)
                n105 = Index Array(array=w607, index=w604) -> (element=w606:string)
                n106 = local write "STATUS"(w606) -> ()
                n107 = call "WSVCAP SHL Host TL RFFE Write - Multiple DUTs - Common Data.vi"("Data Out"=w608, "error in"=w595, "Log (T)"=FALSE) -> ("error out"=w599:errorcluster)  [unwired: 12 in]
                n108 = call "Delay.vi"("milliseconds to wait"=u32 10, "error in (no error)"=w599) -> ("error out"=w603:errorcluster)  [unwired: 9 in]
                n109 = call "WS1050 AD7747 READ 36 DUT.vi"("error in"=w603, "Log (T)"=w596, "DUT Mask Mode (All)"=WSVCAP_SHL_I2C_DUT_Mask_Mode_Enum."C3") -> ("error out"=w601:errorcluster, "AD7747 Values"=w602:string[][])  [unwired: 7 in]
                n110 = for {
                  tunnel: w602 -> [w615] mode=indexing
                  tunnel: w601 -> [w616]
                  tunnel: [w616] -> w597
                  tunnel: [w613] -> w605 mode=indexing
                  n111 = Index Array(array=w615, index=5) -> (element=w613:string)
                }
                n112 = Unbundle By Name(w597) -> ("status"=w611:bool)
                n113 = Or(x=w611, y=w610) -> (x .or. y?=w609:bool)
              }
              n114 = Transpose 2D Array(2D array=w570) -> (transposed array=w577:string[][])
              "40V_3" <- w577
            }
            frame #4 {
              # "VPI Testing @ 35V"
              n115 = call "WS1050 Delta C Calculation.vi"("error in (no error)"=w658, "DCap Target(pF)"=w657, "Input"=w660) -> ("error out"=w655:errorcluster, "% Bank DeltaC"=w652:string[], "Delta B1(pF)"=w619:string[])  [unwired: 3 in, 3 out]
              n116 = call "WS1050 Delta C Calculation.vi"("error in (no error)"=w658, "DCap Target(pF)"=w657, "Input"=w659) -> ("error out"=w656:errorcluster, "% Bank DeltaC"=w650:string[], "Delta B1(pF)"=w618:string[])  [unwired: 3 in, 3 out]
              n117 = call "WS1050 Delta C Calculation.vi"("error in (no error)"=w658, "DCap Target(pF)"=w657, "Input"=w651) -> ("error out"=w654:errorcluster, "% Bank DeltaC"=w649:string[], "Delta B1(pF)"=w617:string[])  [unwired: 3 in, 3 out]
              n118 = Merge Errors(w655, w656, w654) -> (w653:errorcluster)
              n119 = case shown="1, Default" w661 {
                tunnel: w653 -> [w690 w698]
                tunnel: [w690 w698] -> w623
                tunnel: w652 -> [w686 w694]
                tunnel: w650 -> [w685 w693]
                tunnel: w649 -> [w684 w692]
                tunnel: w619 -> [w689 w697]
                tunnel: [w689 w697] -> w648
                tunnel: w618 -> [w688 w696]
                tunnel: [w688 w696] -> w647
                tunnel: w617 -> [w687 w695]
                tunnel: [w687 w695] -> w646
                frame 0 {
                  n120 = Build Array(w686, w685, w684) -> (→"% Delta C_T0":string[][])
                }
                frame 1, Default {
                  n121 = Build Array(w694, w693, w692) -> (→"% Delta C":string[][])
                }
              }
              "Total Delta C1(pF)" <- w648
              "Total Delta C2(pF)" <- w647
              "Total Delta C3(pF)" <- w646
              n122 = call "WS1050_51 VPI Header.vi"("VPI Name"="VPI Name", "VPI_Cmd"="VPI_Cmd", "Cmin/Act"=w621, "WS1050/51"=w632, "error in (no error)"=w633) -> ("VPI_1"=w631:string[], "VPI_2"=w629:string[], "VPI Header"=w630:string[], "VPI_3"=w628:string[], "Cmd_3"=w625:string[], "Cmd_1"=w627:string[], "Cmd_2"=w626:string[], "error out"=w624:errorcluster)  [unwired: 3 in]
              n123 = Merge Errors(w624, w623) -> (w622:errorcluster)
              n124 = case shown="False" w638 {
                tunnel: w674 -> [w705 w743]
                tunnel: [w701 w721] -> w642
                tunnel: [w699 w745] -> w673
                tunnel: [w699 w729] -> w672
                tunnel: [w705 w727] -> w671
                tunnel: w668 -> [w707 w744]
                tunnel: [w707 w744] -> w667
                tunnel: w627 -> [_ w742]
                tunnel: w626 -> [_ w736]
                tunnel: w625 -> [_ w731]
                tunnel: [w699 w741] -> w664
                tunnel: w631 -> [w704 w739]
                tunnel: w629 -> [_ w737]
                tunnel: w628 -> [_ w732]
                tunnel: ["" ("string") w726] -> w644
                tunnel: w622 -> [w702 w718]
                frame False {
                  n125 = Array Size(array=w704) -> (size(s)=w703:i32)
                  n126 = for {
                    N: w703 -> [_]
                    tunnel: [w709] -> w700 mode=indexing
                    shift-right: [w708] -> w701
                    shift-left: w702 -> [w708]
                    n127 = for {
                      N: 36 -> [_]
                      tunnel: [""] -> w709 mode=indexing
                    }
                  }
                  n128 = Transpose 2D Array(2D array=w700) -> (transposed array=w699:string[][])
                  n129 = local write "VPI C1"(w699) -> ()
                  n130 = local write "VPI C2"(w699) -> ()
                  n131 = local write "VPI C3"(w699) -> ()
                }
                frame True {
                  w720 = FALSE ("Log (T)")
                  # "Set CP to 35V"
                  n132 = call "WSVCAP SHL Host TL RFFE Write - Multiple DUTs - Common Data.vi"("Data Out"="074820", "error in"=w718, "Log (T)"=w720) -> ("error out"=w716:errorcluster)  [unwired: 12 in]
                  n133 = call "Delay.vi"("milliseconds to wait"=u32 10, "error in (no error)"=w716) -> ("error out"=w722:errorcluster)  [unwired: 9 in]
                  n134 = case shown="3" "CP VPI" {
                    selector: "CP VPI" -> [w750 w755 w760 w764]
                    tunnel: string[] ["07476F", "074776", "074765", "074769", "07477B"] -> [w751 w756 w761 w766]
                    tunnel: [w749 w754 w759 w765] -> w714
                    tunnel: [w747 w752 w757 w762] -> w713
                    tunnel: ["35" ("string") "27.5" ("string") "30.5" ("string") "40.25" ("string")] -> w726
                    tunnel: w722 -> [w747 w752 w757 w762]
                    frame 0, Default {
                      n135 = Index Array(array=w751, index=w750) -> (element=w749:string)
                    }
                    frame 2 {
                      n136 = Index Array(array=w756, index=w755) -> (element=w754:string)
                    }
                    frame 3 {
                      n137 = Index Array(array=w761, index=w760) -> (element=w759:string)
                    }
                    frame 1 {
                      n138 = Index Array(array=w766, index=w764) -> (element=w765:string)
                    }
                  }
                  n139 = Array Size(array=w739) -> (size(s)=w746:i32)
                  n140 = call "WSVCAP SHL Host TL RFFE Write - Multiple DUTs - Common Data.vi"("Data Out"=w714, "error in"=w713, "Log (T)"=w720) -> ("error out"=w725:errorcluster)  [unwired: 12 in]
                  n141 = for {
                    N: w746 -> [_]
                    tunnel: w742 -> [w831]
                    tunnel: w743 -> [w829]
                    tunnel: [w828] -> w735
                    tunnel: [w826] -> w740 mode=indexing
                    tunnel: w739 -> [w825]
                    tunnel: w725 -> [w814]
                    tunnel: [w816] -> w724
                    i -> [w824]
                    stop <- w828 stop-if-true
                    n142 = Index Array(array=w831, index=w824) -> (element=w827:string)
                    n143 = Index Array(array=w825, index=w824) -> (element=w823:string)
                    n144 = local write "STATUS"(w823) -> ()
                    n145 = call "WSVCAP SHL Host TL RFFE Write - Multiple DUTs - Common Data.vi"("Data Out"=w827, "error in"=w814, "Log (T)"=FALSE) -> ("error out"=w822:errorcluster)  [unwired: 12 in]
                    n146 = call "Delay.vi"("milliseconds to wait"=u32 10, "error in (no error)"=w822) -> ("error out"=w818:errorcluster)  [unwired: 9 in]
                    n147 = call "WS1050 AD7747 READ 36 DUT.vi"("error in"=w818, "Log (T)"=FALSE, "DUT Mask Mode (All)"=WSVCAP_SHL_I2C_DUT_Mask_Mode_Enum."C1") -> ("error out"=w820:errorcluster, "AD7747 Values"=w819:string[][])  [unwired: 7 in]
                    n148 = for {
                      tunnel: [w834] -> w826 mode=indexing
                      tunnel: w820 -> [w833]
                      tunnel: [w833] -> w816
                      tunnel: w819 -> [w832] mode=indexing
                      n149 = Index Array(array=w832, index=1) -> (element=w834:string)
                    }
                    n150 = Unbundle By Name(w816) -> ("status"=w830:bool)
                    n151 = Or(x=w830, y=w829) -> (x .or. y?=w828:bool)
                  }
                  n152 = Transpose 2D Array(2D array=w740) -> (transposed array=w745:string[][])
                  "VPI C1" <- w745
                  n153 = Array Size(array=w737) -> (size(s)=w738:i32)
                  n154 = for {
                    N: w738 -> [_]
                    tunnel: w736 -> [w808]
                    tunnel: w735 -> [w806]
                    tunnel: [w805] -> w728
                    tunnel: [w803] -> w734 mode=indexing
                    tunnel: w737 -> [w802]
                    tunnel: w724 -> [w791]
                    tunnel: [w793] -> w723
                    i -> [w801]
                    stop <- w805 stop-if-true
                    n155 = Index Array(array=w808, index=w801) -> (element=w804:string)
                    n156 = Index Array(array=w802, index=w801) -> (element=w800:string)
                    n157 = call "WSVCAP SHL Host TL RFFE Write - Multiple DUTs - Common Data.vi"("Data Out"=w804, "error in"=w791, "Log (T)"=FALSE) -> ("error out"=w799:errorcluster)  [unwired: 12 in]
                    n158 = local write "STATUS"(w800) -> ()
                    n159 = call "Delay.vi"("milliseconds to wait"=u32 10, "error in (no error)"=w799) -> ("error out"=w795:errorcluster)  [unwired: 9 in]
                    n160 = call "WS1050 AD7747 READ 36 DUT.vi"("error in"=w795, "Log (T)"=FALSE, "DUT Mask Mode (All)"=WSVCAP_SHL_I2C_DUT_Mask_Mode_Enum."C2") -> ("error out"=w797:errorcluster, "AD7747 Values"=w796:string[][])  [unwired: 7 in]
                    n161 = for {
                      tunnel: [w811] -> w803 mode=indexing
                      tunnel: w797 -> [w810]
                      tunnel: [w810] -> w793
                      tunnel: w796 -> [w809] mode=indexing
                      n162 = Index Array(array=w809, index=3) -> (element=w811:string)
                    }
                    n163 = Unbundle By Name(w793) -> ("status"=w807:bool)
                    n164 = Or(x=w807, y=w806) -> (x .or. y?=w805:bool)
                  }
                  n165 = Transpose 2D Array(2D array=w734) -> (transposed array=w741:string[][])
                  "VPI C2" <- w741
                  n166 = Array Size(array=w732) -> (size(s)=w733:i32)
                  n167 = for {
                    N: w733 -> [_]
                    tunnel: w731 -> [w785]
                    tunnel: w728 -> [w783]
                    tunnel: [w782] -> w727
                    tunnel: [w780] -> w730 mode=indexing
                    tunnel: w732 -> [w779]
                    tunnel: w723 -> [w768]
                    tunnel: [w770] -> w721
                    i -> [w778]
                    stop <- w782 stop-if-true
                    n168 = Index Array(array=w785, index=w778) -> (element=w781:string)
                    n169 = Index Array(array=w779, index=w778) -> (element=w777:string)
                    n170 = call "WSVCAP SHL Host TL RFFE Write - Multiple DUTs - Common Data.vi"("Data Out"=w781, "error in"=w768, "Log (T)"=FALSE) -> ("error out"=w776:errorcluster)  [unwired: 12 in]
                    n171 = local write "STATUS"(w777) -> ()
                    n172 = call "Delay.vi"("milliseconds to wait"=u32 10, "error in (no error)"=w776) -> ("error out"=w772:errorcluster)  [unwired: 9 in]
                    n173 = call "WS1050 AD7747 READ 36 DUT.vi"("error in"=w772, "Log (T)"=FALSE, "DUT Mask Mode (All)"=WSVCAP_SHL_I2C_DUT_Mask_Mode_Enum."C3") -> ("error out"=w774:errorcluster, "AD7747 Values"=w773:string[][])  [unwired: 7 in]
                    n174 = for {
                      tunnel: [w788] -> w780 mode=indexing
                      tunnel: w774 -> [w787]
                      tunnel: [w787] -> w770
                      tunnel: w773 -> [w786] mode=indexing
                      n175 = Index Array(array=w786, index=5) -> (element=w788:string)
                    }
                    n176 = Unbundle By Name(w770) -> ("status"=w784:bool)
                    n177 = Or(x=w784, y=w783) -> (x .or. y?=w782:bool)
                  }
                  n178 = Transpose 2D Array(2D array=w730) -> (transposed array=w729:string[][])
                  "VPI C3" <- w729
                }
              }
              n179 = Insert Into Array(array=w663, new element=w630) -> (w662:string[])  [unwired: 1 in]
              n180 = case shown="True" w643 {
                tunnel: w642 -> [w676 w681]
                tunnel: [w677 w680] -> w641
                frame False {
                  n181 = call "WSVCAP SHL Host TL RFFE Write - Multiple DUTs - Common Data.vi"("Data Out"="074820", "error in"=w676, "Log (T)"=FALSE) -> ("error out"=w677:errorcluster)  [unwired: 12 in]
                }
                frame True {
                  n182 = call "WSVCAP SHL Host TL RFFE Write - Multiple DUTs - Common Data.vi"("Data Out"="074800", "error in"=w681, "Log (T)"=FALSE) -> ("error out"=w680:errorcluster)  [unwired: 12 in]
                }
              }
              n183 = call "Delay.vi"("milliseconds to wait"=u32 0, "error in (no error)"=w641) -> ("error out"=w640:errorcluster)  [unwired: 9 in]
            }
            frame #5 {
              # "VSA Testing"
              n184 = case shown="False" w837 {
                tunnel: w875 -> [w887 w901]
                tunnel: [w886 w900] -> w850
                tunnel: [w891 w907] -> w866
                tunnel: w867 -> [w891 w906]
                tunnel: [w888 w904] -> w855
                tunnel: [w888 w903] -> w852
                tunnel: [w888 w902] -> w849
                tunnel: [w889 w905] -> w856
                frame False {
                  n185 = for {
                    tunnel: dbl[] [0.0, 0.0, 0.0] -> [w896] mode=indexing
                    tunnel: [w895] -> w889 mode=indexing
                    tunnel: [w892] -> w888 mode=indexing
                    shift-right: [w893] -> w886
                    shift-left: w887 -> [w893]
                    n186 = Number To Fractional String(number=w896) -> (F-format string=w897:string)  [unwired: 3 in]
                    n187 = for {
                      N: 36 -> [_]
                      tunnel: w897 -> [w899]
                      tunnel: [w899] -> w895 mode=indexing
                      tunnel: [""] -> w892 mode=indexing
                    }
                  }
                }
                frame True {
                  n188 = for {
                    tunnel: "VSA Voltage(V)" -> [w931] mode=indexing
                    tunnel: [w935] -> w907
                    tunnel: w906 -> [w933]
                    tunnel: [w932] -> w904 mode=indexing
                    tunnel: [w919] -> w903 mode=indexing
                    tunnel: [w928] -> w905 mode=indexing
                    tunnel: [w913] -> w902 mode=indexing
                    tunnel: w901 -> [w912]
                    tunnel: [w911] -> w900
                    w910 = FALSE ("Log (T)")
                    w927 = u16 0 items=["Voltage", "Current"] ("Source Mode  (0: Voltage)")
                    n189 = call "Ke2400 Configure Output.vi"("Source Mode  (0: Voltage)"=w927, "error in (no error)"=w912, "Compliance  Level (0.1)"=0.1, "Output Level (0)"=w931, "VISA resource name"=w933) -> ("error out"=w939:errorcluster, "VISA resource name out"=w937:refnum<visa-resource-name>)  [unwired: 5 in]
                    n190 = call "Ke2400 Enable.vi"("error in (no error)"=w939, "ON/OFF"=TRUE ("Enable Output (T: Enable)"), "VISA resource name"=w937) -> ("error out"=w940:errorcluster, "VISA resource name out"=w935:refnum<visa-resource-name>)  [unwired: 7 in]
                    n191 = call "Delay.vi"("milliseconds to wait"=u32 10, "error in (no error)"=w940) -> ("error out"=w926:errorcluster)  [unwired: 9 in]
                    n192 = call "WS1050 AD7747 READ 36 DUT.vi"("error in"=w926, "Log (T)"=w910, "DUT Mask Mode (All)"=WSVCAP_SHL_I2C_DUT_Mask_Mode_Enum."C1") -> ("error out"=w923:errorcluster, "AD7747 Values"=w925:string[][])  [unwired: 7 in]
                    n193 = for {
                      tunnel: w925 -> [w951] mode=indexing
                      tunnel: [w952] -> w932 mode=indexing
                      tunnel: w923 -> [w950]
                      tunnel: [w950] -> w922
                      n194 = Index Array(array=w951, index=1) -> (element=w952:string)
                    }
                    n195 = call "WS1050 AD7747 READ 36 DUT.vi"("error in"=w922, "Log (T)"=w910, "DUT Mask Mode (All)"=WSVCAP_SHL_I2C_DUT_Mask_Mode_Enum."C2") -> ("error out"=w920:errorcluster, "AD7747 Values"=w918:string[][])  [unwired: 7 in]
                    n196 = for {
                      tunnel: w918 -> [w946] mode=indexing
                      tunnel: [w947] -> w919 mode=indexing
                      tunnel: w920 -> [w945]
                      tunnel: [w945] -> w917
                      n197 = Index Array(array=w946, index=3) -> (element=w947:string)
                    }
                    n198 = Number To Fractional String(number=w931) -> (F-format string=w930:string)  [unwired: 3 in]
                    n199 = call "WS1050 AD7747 READ 36 DUT.vi"("error in"=w917, "Log (T)"=w910, "DUT Mask Mode (All)"=WSVCAP_SHL_I2C_DUT_Mask_Mode_Enum."C3") -> ("error out"=w915:errorcluster, "AD7747 Values"=w914:string[][])  [unwired: 7 in]
                    n200 = for {
                      tunnel: w914 -> [w942] mode=indexing
                      tunnel: [w943] -> w913 mode=indexing
                      tunnel: w915 -> [w941]
                      tunnel: [w941] -> w911
                      n201 = Index Array(array=w942, index=5) -> (element=w943:string)
                    }
                    n202 = for {
                      N: 36 -> [_]
                      tunnel: w930 -> [w949]
                      tunnel: [w949] -> w928 mode=indexing
                    }
                  }
                  n203 = local write "STATUS"("VSA Testing...." ("STATUS")) -> ()
                }
              }
              n204 = Transpose 2D Array(2D array=w856) -> (transposed array=w854:string[][])
              n205 = Transpose 2D Array(2D array=w855) -> (transposed array=w853:string[][])
              n206 = Transpose 2D Array(2D array=w852) -> (transposed array=w851:string[][])
              n207 = Transpose 2D Array(2D array=w849) -> (transposed array=w848:string[][])
              n208 = call "WS1050_VSA_Convert_Data.vi"("VSA_C3"=w848, "error in (no error)"=w850, "VSA_C2"=w851, "VSA_C1"=w853, "Voltage"=w854) -> ("error out"=w847:errorcluster, "VSA_V3"=w844:string[][], "VSA_V2"=w845:string[][], "VSA_V1"=w846:string[][])  [unwired: 3 in]
              "VSA_V1" <- w846
              "VSA_V2" <- w845
              "VSA_V3" <- w844
              n209 = case shown="True" w837 {
                tunnel: w866 -> [w879 w885]
                tunnel: [w879 w884] -> w865
                tunnel: w847 -> [w878 w883]
                tunnel: [w878 w880] -> w864
                frame False {
                }
                frame True {
                  w881 = u16 0 items=["Voltage", "Current"] ("Source Mode  (0: Voltage)")
                  n210 = call "Ke2400 Configure Output.vi"("Source Mode  (0: Voltage)"=w881, "error in (no error)"=w883, "Output Level (0)"=0.0, "VISA resource name"=w885) -> ("error out"=w880:errorcluster, "VISA resource name out"=w884:refnum<visa-resource-name>)  [unwired: 6 in]
                }
              }
              n211 = call "Delay.vi"("milliseconds to wait"=u32 0, "error in (no error)"=w864) -> ("error out"=w863:errorcluster)  [unwired: 9 in]
            }
            frame #6 {
              # "Handshake Check and EFuse Readback"
              n212 = Or(x=w965, y=w971) -> (x .or. y?=w970:bool)
              n213 = case shown="True" w970 {
                tunnel: w993 -> [w1006 _]
                tunnel: w992 -> [w1005 w1010]
                tunnel: [w1004 w1009] -> w991
                tunnel: w990 -> [w1003 _]
                tunnel: w989 -> [w1002 _]
                tunnel: w988 -> [w1001 _]
                tunnel: [w997 w1012] -> w987
                tunnel: [w996 w1012] -> w982
                tunnel: w955 -> [w995 _]
                tunnel: w976 -> [w994 _]
                frame False {
                  n214 = call "WS1050_36DUT_Handshake Check R1_Record All Regs Ver1.0.vi"("file path (use dialog)"=w1006, "Reg1_Bit Cntrl"="Reg1_Bit Cntrl", "File Name"=w994, "SN"=w1001, "Loop"=w995, "error"=w1005, "Lot #"=w1003, "Wafer #"=w1002) -> ("Pass/Fail"=→"EFuse Readback Status":bool[], "EFuse Read back"=w996:string[], "Status"=w997:string[], "error out"=w1004:errorcluster)  [unwired: 6 in, 2 out]
                  n215 = case shown="1, Default" w995 {
                    tunnel: w996 -> [w1007 w1008]
                    frame 0 {
                      "EFuse RB T0" <- w1007
                    }
                    frame 1, Default {
                      "Current EFuse Read back" <- w1008
                    }
                  }
                  n216 = local write "STATUS"("Hand Shake & EFuse Readback...." ("STATUS")) -> ()
                }
                frame True {
                  n217 = for {
                    N: 36 -> [_]
                    tunnel: [""] -> w1012 mode=indexing
                    tunnel: w1010 -> [w1013]
                    tunnel: [w1013] -> w1009
                  }
                }
              }
              n218 = Build Array(w980, w978, w977) -> (w979:string[])
            }
            frame #7 {
              # "Save Data"
              n219 = Increment(x=w1028) -> (x+1=w1016:i32)
              n220 = local write "STATUS"("Saving Data...." ("STATUS")) -> ()
              n221 = Multiply(x=w1016, y=36) -> (x*y=w1024:i32)
              n222 = Path To String(path=w1032) -> (string=w1031:string)
              n223 = Bundle("Test Program"=w1060, "Comment"=w1059, "Data Out"=w1039, "Data Out"=w1038, "CP Voltage"=w1037, w1036, "% Duty Cycle"=w1035, "CP Voltage"=w1034, "string"=w1033, "Freq(Hz)"=w1022, "Board#"=w1020) -> (w1021:T5)  [unwired: 1 in]
              n224 = case shown="True" w1017 {
                tunnel: w1024 -> [w1067 w1070]
                tunnel: [w1067 w1068] -> w1023
                frame False {
                }
                frame True {
                  n225 = Multiply(x=w1070, y="No of Rows\nFrom Spread Sheet") -> (x*y=w1068:i32)
                }
              }
              n226 = call "WS1050_36 DUT SData Ver1.0.vi"("TMN DC\\CAP Data Log File Path"=w1032, "Lot#"=w1062, "Total Delta C1(pF)"=w1042, "VSA_V1"=w1049, "Wafer#"=w1058, "File Name"=w1026, "Total Delta C2(pF)"=w1041, "error in"=w1065, "TP/Comment"=w1021, "EFuse"=w1052, "Data Output C3"=w1043, "Temperature"=w1047, "VSA_V2"=w1050, "VPI C3"=w1045, "Data Output C1"=w1055, "VPI C2"=w1044, "SN"=w1063, "R/W Status"=w1061, "Cap Header"=w1046, "HD/Cycles Completed"="HD/Cycles Completed", "Data Output C2"=w1015, "VSA_V3"=w1048, "Current"=w1054, "VPI C1"=w1053, "Total Delta C3(pF)"=w1040) -> ("error out"=w1064:errorcluster)  [unwired: 2 in]
              n227 = Concatenate Strings(w1031, "\\" ("string"), w1026, "_Multi Socket Data.csv" ("string")) -> (w1030:string)
            }
            frame #8 {
              n228 = case shown="True" "Plot Delta Cmin" {
                tunnel: w1079 -> [w1088 w1103]
                tunnel: [w1088 w1099] -> w1078
                tunnel: w1077 -> [_ w1095]
                tunnel: w1075 -> [_ w1093]
                frame False {
                }
                frame True {
                  n229 = String To Path(string=w1095) -> (path=w1094:path)
                  n230 = call "Delay.vi"("milliseconds to wait"=u32 50, "error in (no error)"=w1103) -> ("error out"=w1102:errorcluster)  [unwired: 9 in]
                  n231 = call "36DUT Plot From Spread Sheet.vi"("Plot"="Plot", "No of Rows"=w1093, "error in (no error)"=w1102, "Bank"="Bank1", "file path (dialog if empty)"=w1094) -> ("error out"=w1097:errorcluster, "Delta C_Min Plot"=→"Plot_1":dbl[][])  [unwired: 5 in]
                  n232 = call "36DUT Plot From Spread Sheet.vi"("Plot"="Plot", "No of Rows"=w1093, "error in (no error)"=w1097, "Bank"="Bank2", "file path (dialog if empty)"=w1094) -> ("error out"=w1098:errorcluster, "Delta C_Min Plot"=→"Plot_2":dbl[][])  [unwired: 5 in]
                  n233 = call "36DUT Plot From Spread Sheet.vi"("Plot"="Plot", "No of Rows"=w1093, "error in (no error)"=w1098, "Bank"="Bank3", "file path (dialog if empty)"=w1094) -> ("error out"=w1099:errorcluster, "Delta C_Min Plot"=→"Plot_3":dbl[][])  [unwired: 5 in]
                }
              }
              n234 = Increment(x=w1072) -> (x+1=w1071:i32)
              "No of HD/Cycle\nCompleted" <- w1071
              n235 = Get Date/Time In Seconds() -> (seconds since 1Jan1904=w1081:timestamp)
              n236 = Get Date/Time String(seconds (now)=w1081, want seconds? (F)=TRUE) -> (date string=→"date string":string, time string=→"Previous Time":string)  [unwired: 1 in]
              n237 = local write "RB Reg for HD/Cycle"(string[] []) -> ()
              n238 = Greater Or Equal?(x=w1071, y=w1074) -> (x >= y?=w1085:bool)
            }
          }
          n239 = call "Delay.vi"("milliseconds to wait"=u32 10, "error in (no error)"=w219) -> ("error out"=w220:errorcluster)  [unwired: 9 in]
          n240 = Compound Arithmetic op=OR(w371, w291) -> (w320:bool)
          "Loop \ncompleted" <- w163
        }
        n241 = local write "No of HD/Cycle\nCompleted"(u64 0 ("No of HD/Cycle\nCompleted")) -> ()
        n242 = Unbundle By Name(w145) -> ("status"=w151:bool)
        n243 = Compound Arithmetic op=OR(w151, w149) -> (w135:bool)
      }
      n244 = VISA Write(VISA resource name=w67, write buffer="SOUR:FUNC VOLT;VOLT:MODE FIX;RANG 100;LEV 0.0;:SENS:FUNC \"CURR\";CURR:PROT 60E-3;RANG 100E-3;:OUTP ON", error in (no error)=w53) -> (VISA resource name out=w66:refnum<visa-resource-name>, error out=w32:errorcluster)  [unwired: 1 out]
    }
  }
  "Ke2000 Out" <- w22
  "PS1 Out" <- w21
  "Ke2400 Out" <- w16
  "error out" <- w15
  "STATUS" <- "Idle...." ("STATUS")
